vi "启动.vi"() -> ()   [LabVIEW 2014]
doc: "This example uses VI Server to display a splash screen for your main application while all its subVIs load into memory. This is useful if you have a large application that takes a while to load, because the splash screen can display your company information, along with an indicator displaying the load status.\n\nThe VI uses a hidden string indicator in conjuction with a horizontal bar control to achieve the desired user interface."
panel:
  out "Current Status":string
  out "String":string
  out "Slide":u8(slide) scale=0.0..50.0
  # "Version: C.1.0\n--\n南京天创智能所有, 2015"
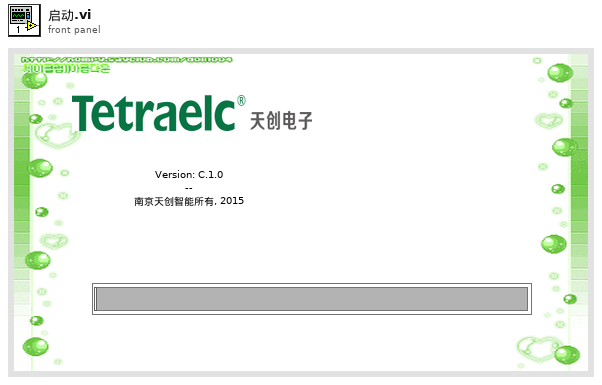
[diagram p1: front panel]
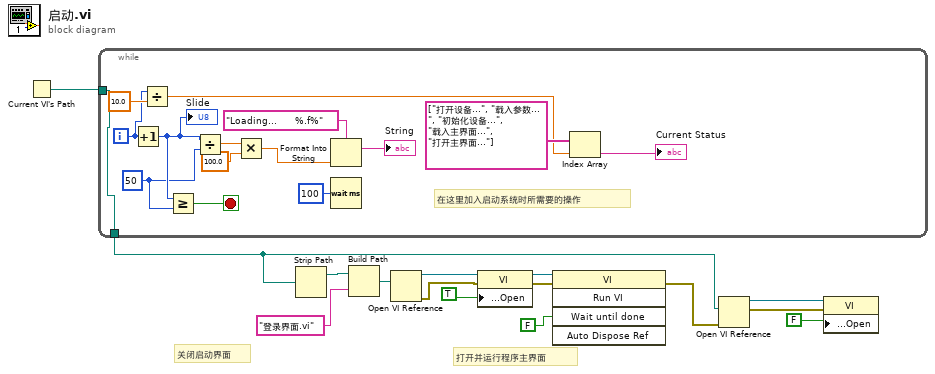
[diagram p0: block diagram]
diagram:
  # "打开并运行程序主界面"
  # "关闭启动界面"
  n1 = Current VI's Path() -> (path=w5:path)
  n2 = while {
    tunnel: w5 -> [w23]
    tunnel: [w23] -> w3
    i -> [w17]
    stop <- w28 stop-if-true
    w25 = 50 ("y")
    # "在这里加入启动系统时所需要的操作"
    n3 = Increment(x=w17) -> (x+1=w27:i32)
    "Slide" <- w27
    n4 = Divide(x=w17, y=10.0) -> (x/y=w16:dbl)
    n5 = Greater Or Equal?(x=w27, y=w25) -> (x >= y?=w28:bool)
    n6 = Divide(x=w27, y=w25) -> (x/y=w26:dbl)
    n7 = Multiply(x=w26, y=100.0) -> (x*y=w22:dbl)
    n8 = Format Into String(format string="Loading...      %.f%", w22) -> (resulting string=→"String":string)  [unwired: 2 in, 1 out]
    n9 = Wait (ms)(milliseconds to wait=u32 100) -> ()  [unwired: 1 out]
    n10 = Index Array(array=string[] ["打开设备...", "载入参数...", "初始化设备...", "载入主界面...", "打开主界面..."], index=w16) -> (element=→"Current Status":string)
  }
  n11 = Strip Path(path=w3) -> (stripped path=w4:path)  [unwired: 1 out]
  n12 = Build Path(base path=w4, name or relative path="登录界面.vi" ("名称或相对路径")) -> (appended path=w6:path)
  n13 = Open VI Reference(vi path=w6) -> (vi reference=w7:refnum<vi>, error out=w8:errorcluster)  [unwired: 5 in]
  n14 = property on="Property Node" class="VI"(reference=w7, error in=w8, "Front Panel Window:Open"=TRUE) -> (reference out=w10:refnum<vi>, error out=w11:errorcluster)
  n15 = invoke class="VI" method="Run VI"(reference=w10, error in=w11, "Wait until done"=FALSE) -> (error out=w1:errorcluster)  [unwired: 2 in, 4 out]
  n16 = Open VI Reference(vi path=w3, error in (no error)=w1) -> (vi reference=w15:refnum<vi>, error out=w13:errorcluster)  [unwired: 4 in]
  n17 = property on="Property Node" class="VI"(reference=w15, error in=w13, "Front Panel Window:Open"=FALSE) -> ()  [unwired: 2 out]
